vi "Set which board.vi"(8 "error in (no error)":errorcluster, 10 "which board":T1, 11 "Assembly Line Input in":refnum<class "Assembly Line Input.lvclass">) -> (0 "error out":errorcluster, 3 "Assembly Line Input out":refnum<class "Assembly Line Input.lvclass">)   [LabVIEW 2018, in "Assembly Line Input.lvclass"]
uses:
  Assembly Line Input.lvclass
  Common/Board Type Enum.ctl
  Assembly Line Input.lvclass/Assembly Line Input.ctl
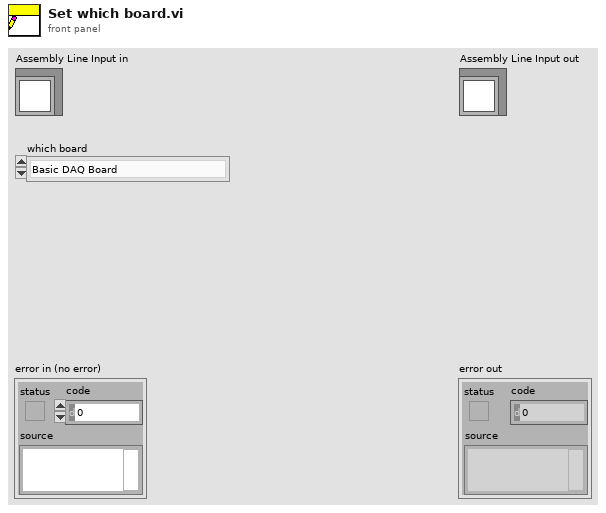
[diagram p1: front panel]
types:
  T1 = typedef "Board Type Enum.ctl" = enum16{"Basic DAQ Board", "Elite DAQ Board", "GPIB Board"}
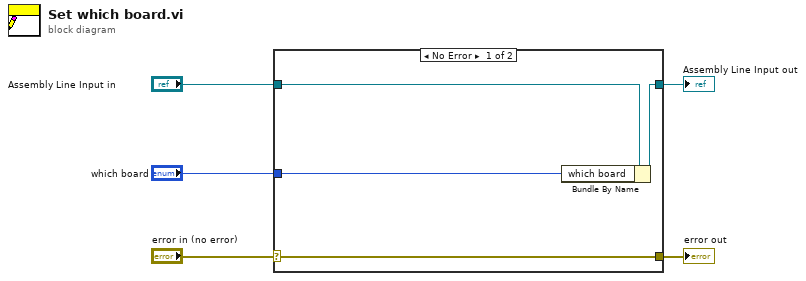
[diagram p0: block diagram]
diagram:
  n1 = case shown="No Error" "error in (no error)" {
    selector: "error in (no error)" -> [w9 w10]
    tunnel: [w9 w10] -> w4
    tunnel: [w7 w11] -> w2
    tunnel: "Assembly Line Input in" -> [w8 w11]
    tunnel: "which board" -> [w6 _]
    frame No Error {
      n2 = Bundle By Name(cluster=w8, "which board"=w6) -> (w7:refnum<class "Assembly Line Input.lvclass">)
    }
    frame Error {
    }
  }
  "error out" <- w4
  "Assembly Line Input out" <- w2
